vi "STICK_init.vi"(2 "error in (no error)":errorcluster, 3 "VISA Refnum in":refnum<visa-resource-name>="COM4") -> (0 "error out":errorcluster, 1 "VISA Refnum out":refnum<visa-resource-name>)   [LabVIEW 2014]
uses:
  <vilib>/Instr/_visa.llb/VISA Configure Serial Port (Instr).vi
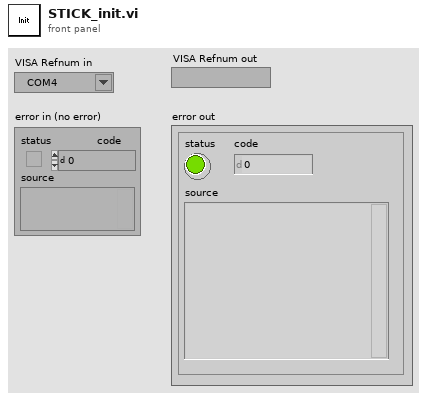
[diagram p1: front panel]
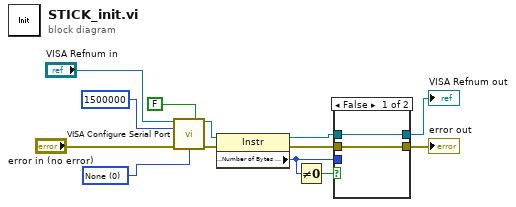
[diagram p0: block diagram]
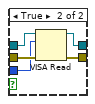
[diagram p2: hidden frame]
diagram:
  w13 = u16 0 items=["None", "XON/XOFF", "RTS/CTS", "XON/XOFF & RTS/CTS", "DTR/DSR", "XON/XOFF & DTR/DSR"] ("flow control (0:none)")
  n1 = call-poly "VISA Configure Serial Port"("VISA resource name"="VISA Refnum in", "Enable Termination\nChar (T)"=FALSE ("Enable Termination\nChar (T)"), "baud rate (9600)"=u32 1500000, "error in (no error)"="error in (no error)", "flow control (0:none)"=w13) -> ("VISA resource name out"=w6:refnum<visa-resource-name>, "error out"=w5:errorcluster)  [unwired: 9 in]
  n2 = property class="Instr"(reference=w6, error in=w5) -> (reference out=w7:refnum<visa-resource-name>, error out=w8:errorcluster, "Serial Settings:Number of Bytes at Serial Port"=w10:u32)
  n3 = Not Equal To 0?(x=w10) -> (x != 0?=w9:bool)
  n4 = case shown="False" w9 {
    tunnel: w7 -> [w15 w20]
    tunnel: w8 -> [w14 w19]
    tunnel: w10 -> [_ w18]
    tunnel: [w15 w17] -> w11
    tunnel: [w14 w16] -> w12
    frame False {
    }
    frame True {
      n5 = VISA Read(VISA resource name=w20, byte count=w18, error in (no error)=w19) -> (VISA resource name out=w17:refnum<visa-resource-name>, error out=w16:errorcluster)  [unwired: 2 out]
    }
  }
  "VISA Refnum out" <- w11
  "error out" <- w12
